vi "Prime BSI Set Get ROI.vi"(0 "Notifier In":refnum<notifier>, 5 "PVCam Actions":T3, 7 "Camera Ref":refnum<k24>, 11 "Error In":errorcluster, 13 "Image Ref":T1) -> (4 "Notifier Out":refnum<notifier>, 8 "PVCam Cluster":T2, 15 "Error Out":errorcluster)   [LabVIEW 2020]
uses:
  Prime BSI Type Defs/Prime BSI Actions.ctl
  C:/Users/Public/Documents/Photometrics/PMQI-LabViewSamples BETA/Examples/2020/Dependencies/PVCamNET.dll
  Public/Documents/Photometrics/PMQI-LabViewSamples BETA/Examples/2020/Dependencies/PVCamNET.dll
  Prime BSI Type Defs/Prime BSI Notifier Element.ctl
  Prime BSI Type Defs/Prime BSI Parameters.ctl
  Prime BSI Type Defs/Prime BSI Parameter List.ctl
  Prime BSI Type Defs/Prime BSI ROI.ctl
  <vilib>/vision/Image Controls.llb/IMAQ Image.ctl
  Camera Controls/Camera IMAQ Key Info.ctl
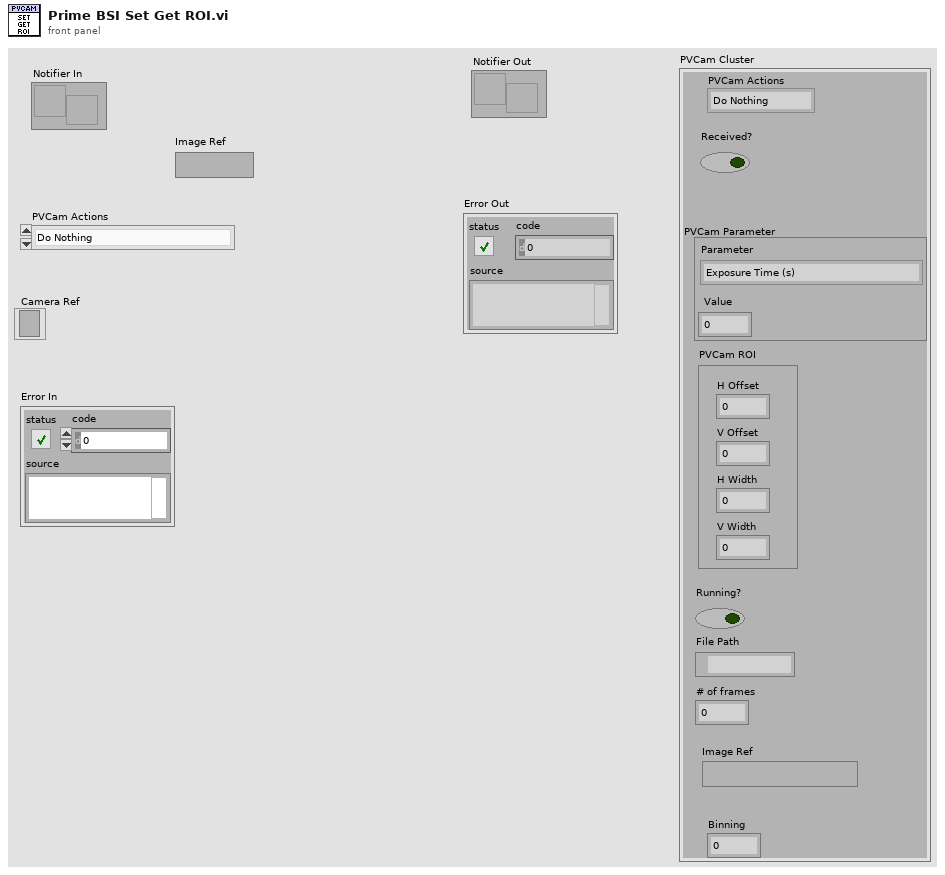
[diagram p1: front panel]
types:
  T1 = typedef "IMAQ Image.ctl" = refnum<image>
  T2 = typedef "Prime BSI Notifier Element.ctl" = cluster{"PVCam Actions":T3, "Received?":bool, "PVCam Parameter":T4, "PVCam ROI":T6, "Running?":bool, "File Path":path, "# of frames":u32, "Image Ref":T1, "Binning":i32}
  T3 = typedef "Prime BSI Actions.ctl" = enum16{"Do Nothing", "Preview", "Record", "Abort", "Record Settings", "Set Parameter", "Get Parameter", "Set ROI", "Get ROI", "Status", "Quit"}
  T4 = typedef "Prime BSI Parameters.ctl" = cluster{"Parameter":T5, "Value":dbl}
  T5 = typedef "Prime BSI Parameter List.ctl" = enum16{"Exposure Time (s)", "Binning"}
  T6 = typedef "Prime BSI ROI.ctl" = cluster{"H Offset":i32, "V Offset":i32, "H Width":i32, "V Width":i32}
  T7 = typedef "Camera IMAQ Key Info.ctl" = cluster{"Frame":u32, "Sensor Height":i32, "Sensor Width":i32, "ROI Height":i32, "ROI Width":i32, "ROI Enable?":bool, "Bit per Pixel":u8}
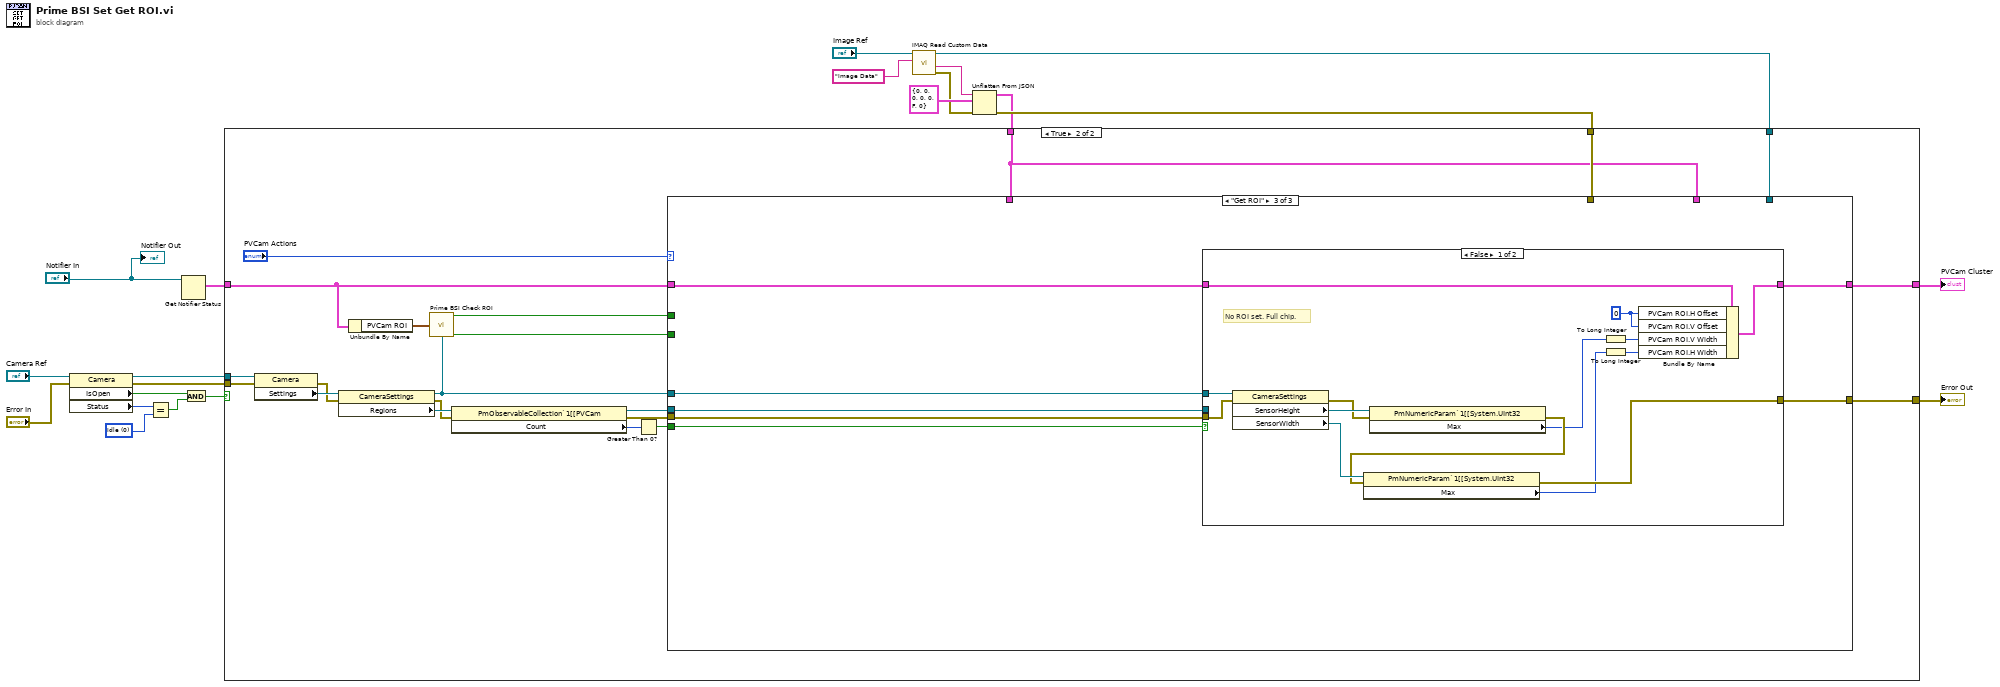
[diagram p0: block diagram]
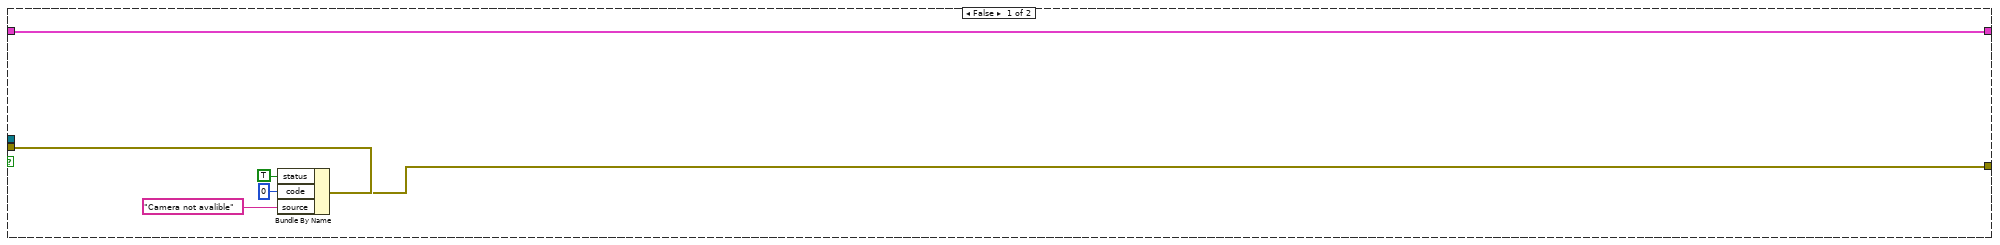
[diagram p2: hidden frame]
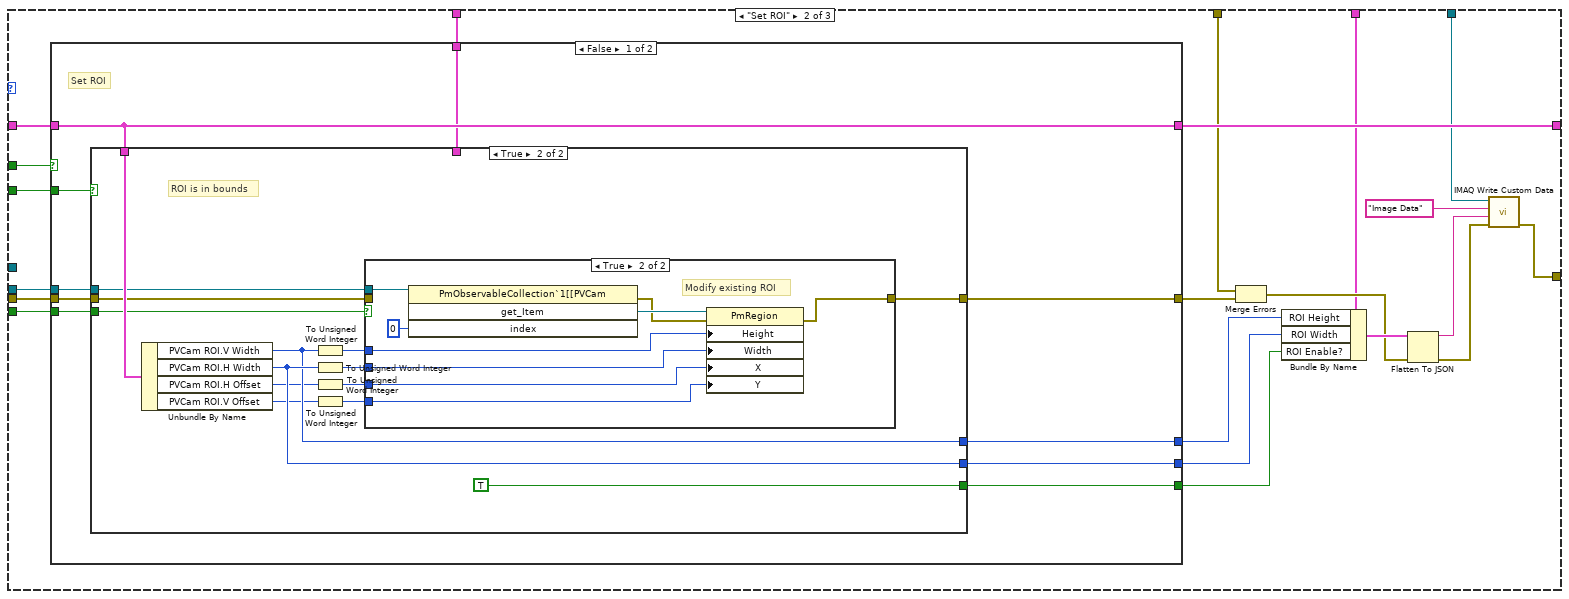
[diagram p4: hidden frame]
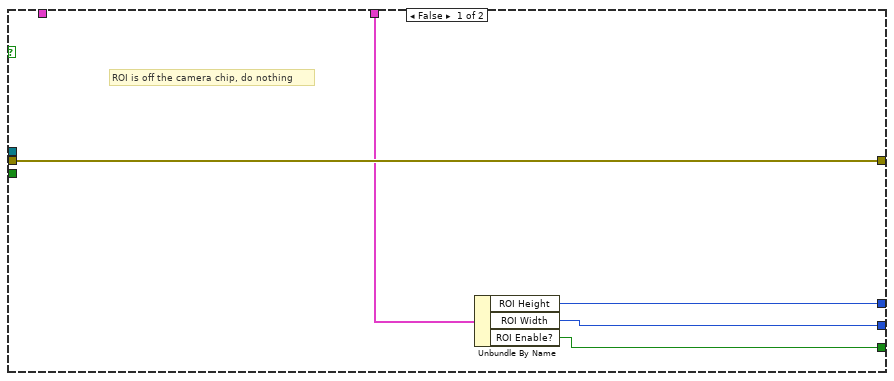
[diagram p5: hidden frame]
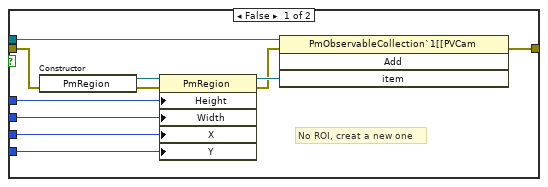
[diagram p6: hidden frame]
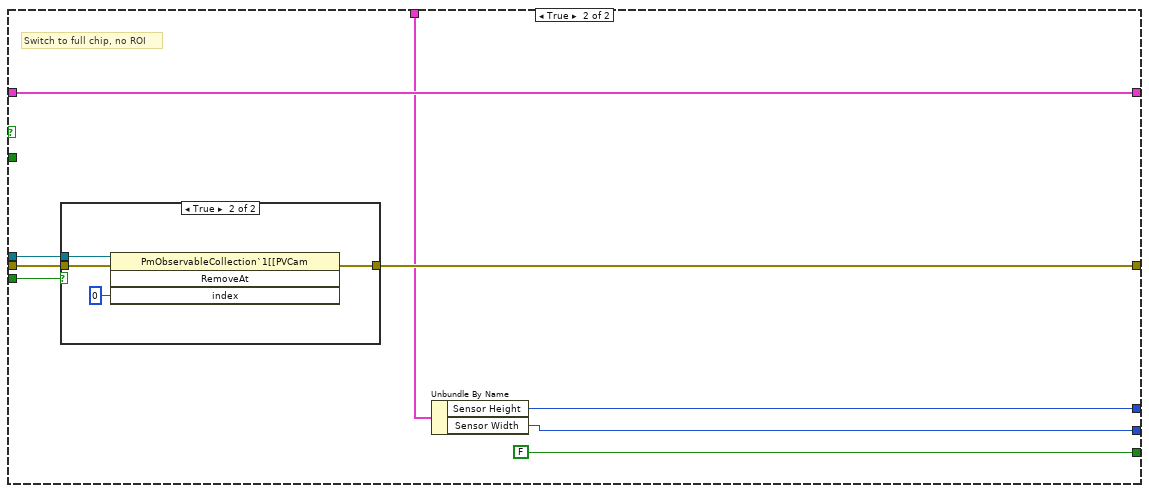
[diagram p7: hidden frame]
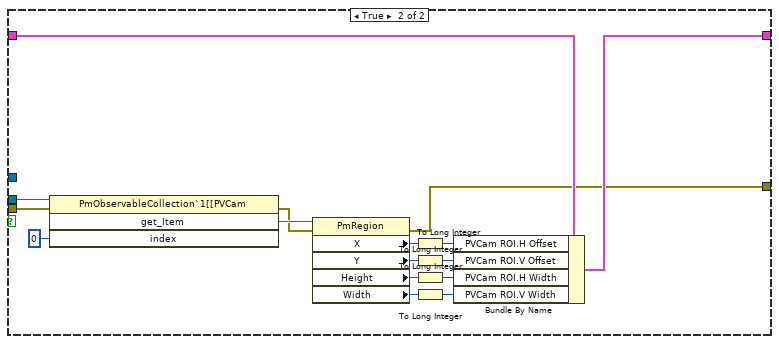
[diagram p9: hidden frame]
diagram:
  w20 = 0 items=["Idle", "Capturing"] ("Status")
  n1 = property class="Camera"(reference="Camera Ref", error in="Error In") -> (reference out=w14:refnum<k24>, error out=w13:errorcluster, "IsOpen"=w19:bool, "Status"=w21:i32)
  n2 = Equal?(x=w21, y=w20) -> (x = y?=w18:bool)
  n3 = Get Notifier Status(notifier="Notifier In") -> (current notification=w10:T2)  [unwired: 1 in, 4 out]
  n4 = And(x=w19, y=w18) -> (x .and. y?=w15:bool)
  n5 = call "IMAQ Read Custom Data"("Key"="Image Data", "Image"="Image Ref") -> ("error out"=w4:errorcluster, "Custom Data Out"=w6:string, "Image (duplicate)"=w3:T1)  [unwired: 7 in]
  n6 = Unflatten From JSON(JSON string=w6, type and defaults=T7 {"Frame"=0, "Sensor Height"=0, "Sensor Width"=0, "ROI Height"=0, "ROI Width"=0, "ROI Enable?"=FALSE, "Bit per Pixel"=0} ("Camera IMAQ Key Info"), error in (no error)=w4) -> (value=w1:T7, error out=w2:errorcluster)  [unwired: 4 in]
  n7 = case shown="True" w15 {
    tunnel: w14 -> [_ w48]
    tunnel: w13 -> [w27 w47]
    tunnel: [w23 w46] -> w12
    tunnel: [w22 w44] -> w11
    tunnel: w10 -> [w22 w41]
    tunnel: w3 -> [_ w40]
    tunnel: w2 -> [_ w39]
    tunnel: w1 -> [_ w37]
    frame False {
      n8 = Bundle By Name(cluster=w27, "status"=TRUE, "code"=0, "source"="Camera not avalible") -> (w23:errorcluster)
    }
    frame True {
      n9 = property class="Camera"(reference=w48, error in=w47) -> (error out=w42:errorcluster, "Settings"=w43:refnum<k24>)  [unwired: 1 out]
      n10 = property class="CameraSettings"(reference=w43, error in=w42) -> (reference out=w28:refnum<k24>, error out=w32:errorcluster, "Regions"=w33:refnum<k24>)
      n11 = Unbundle By Name(w41) -> ("PVCam ROI"=w38:T6)
      n12 = call "Prime BSI Check ROI.vi"("PVCam ROI"=w38, "Cam Settings Ref"=w28) -> ("Full Chip?"=w36:bool, "ROI In Bounds?"=w35:bool)  [unwired: 12 in]
      n13 = property class="PmObservableCollection`1[[PVCam"(reference=w33, error in=w32) -> (reference out=w29:refnum<k24>, error out=w30:errorcluster, "Count"=w34:i32)
      n14 = Greater Than 0?(x=w34) -> (x > 0?=w31:bool)
      n15 = case shown="\"Get ROI\"" "PVCam Actions" {
        tunnel: [w49 w66 w139] -> w46
        tunnel: w41 -> [w50 w70 w141]
        tunnel: [w50 w65 w140] -> w44
        tunnel: w36 -> [_ w71 _]
        tunnel: w40 -> [_ w61 _]
        tunnel: w39 -> [_ w58 _]
        tunnel: w37 -> [_ w56 _]
        tunnel: w37 -> [_ w55 _]
        tunnel: w35 -> [_ w54 _]
        tunnel: w31 -> [_ w51 w138]
        tunnel: w30 -> [w49 w53 w137]
        tunnel: w29 -> [_ w52 w136]
        tunnel: w28 -> [_ _ w135]
        frame Default {
        }
        frame "Set ROI" {
          n16 = case shown="False" w71 {
            tunnel: w51 -> [w73 w129]
            tunnel: w52 -> [w72 w128]
            tunnel: w53 -> [w74 w127]
            tunnel: [w81 w126] -> w59
            tunnel: w70 -> [w80 w124]
            tunnel: [w80 w124] -> w65
            tunnel: [w78 w122] -> w63
            tunnel: [w79 FALSE ("ROI Enable?")] -> w64
            tunnel: [w77 w121] -> w62
            tunnel: w56 -> [w75 w123]
            tunnel: w54 -> [w76 _]
            frame False {
              # "Set ROI"
              n17 = case shown="True" w76 {
                tunnel: w74 -> [w86 w88]
                tunnel: [w86 w87] -> w81
                tunnel: w80 -> [_ w100]
                tunnel: [w84 TRUE ("ROI Enable?")] -> w79
                tunnel: [w82 w98] -> w78
                tunnel: [w83 w97] -> w77
                tunnel: w75 -> [w85 _]
                tunnel: w73 -> [_ w90]
                tunnel: w72 -> [_ w89]
                frame False {
                  # "ROI is off the camera chip, do nothing"
                  n18 = Unbundle By Name(w85) -> ("ROI Height"=w83:i32, "ROI Width"=w82:i32, "ROI Enable?"=w84:bool)
                }
                frame True {
                  # "ROI is in bounds"
                  n19 = Unbundle By Name(w100) -> ("PVCam ROI.V Width"=w97:i32, "PVCam ROI.H Width"=w98:i32, "PVCam ROI.H Offset"=w96:i32, "PVCam ROI.V Offset"=w95:i32)
                  n20 = To Unsigned Word Integer(number=w97) -> (unsigned 16bit integer=w93:u16)
                  n21 = To Unsigned Word Integer(number=w98) -> (unsigned 16bit integer=w92:u16)
                  n22 = To Unsigned Word Integer(number=w96) -> (unsigned 16bit integer=w91:u16)
                  n23 = To Unsigned Word Integer(number=w95) -> (unsigned 16bit integer=w94:u16)
                  n24 = case shown="True" w90 {
                    tunnel: w94 -> [w110 w114]
                    tunnel: w93 -> [w109 w117]
                    tunnel: w92 -> [w108 w116]
                    tunnel: w91 -> [w107 w115]
                    tunnel: w89 -> [w106 w120]
                    tunnel: w88 -> [w104 _]
                    tunnel: [w101 w112] -> w87
                    frame False {
                      # "No ROI, creat a new one"
                      n25 = constructor class="PmRegion"(error in=w104) -> (reference out=w111:refnum<k24>, error out=w103:errorcluster)  [unwired: 2 in, 1 out]
                      n26 = property class="PmRegion"(reference=w111, error in=w103, "Height"=w109, "Width"=w108, "X"=w107, "Y"=w110) -> (reference out=w105:refnum<k24>, error out=w102:errorcluster)
                      n27 = invoke class="PmObservableCollection`1[[PVCam" method="Add"(reference=w106, error in=w102, "item"=w105) -> (error out=w101:errorcluster)  [unwired: 1 in, 3 out]
                    }
                    frame True {
                      # "Modify existing ROI"
                      n28 = invoke class="PmObservableCollection`1[[PVCam" method="get_Item"(reference=w120, "index"=0) -> (error out=w113:errorcluster, "get_Item"=w118:refnum<k24>)  [unwired: 2 in, 2 out]
                      n29 = property class="PmRegion"(reference=w118, error in=w113, "Height"=w117, "Width"=w116, "X"=w115, "Y"=w114) -> (error out=w112:errorcluster)  [unwired: 1 out]
                    }
                  }
                }
              }
            }
            frame True {
              # "Switch to full chip, no ROI"
              n30 = case shown="True" w129 {
                tunnel: w128 -> [_ w134]
                tunnel: w127 -> [w130 w133]
                tunnel: [w130 w131] -> w126
                frame False {
                }
                frame True {
                  n31 = invoke class="PmObservableCollection`1[[PVCam" method="RemoveAt"(reference=w134, error in=w133, "index"=0) -> (error out=w131:errorcluster)  [unwired: 1 in, 3 out]
                }
              }
              n32 = Unbundle By Name(w123) -> ("Sensor Height"=w121:i32, "Sensor Width"=w122:i32)
            }
          }
          n33 = Merge Errors(w58, w59) -> (w57:errorcluster)
          n34 = Bundle By Name(cluster=w55, "ROI Height"=w62, "ROI Width"=w63, "ROI Enable?"=w64) -> (w67:T7)
          n35 = Flatten To JSON(anything=w67, error in (no error)=w57) -> (JSON string=w68:string, 11:w69:errorcluster)  [unwired: 1 in]
          n36 = call "IMAQ Write Custom Data"("error in (no error)"=w69, "Custom Data In"=w68, "Key"="Image Data", "Image"=w61) -> ("error out"=w66:errorcluster)  [unwired: 6 in, 1 out]
        }
        frame "Get ROI" {
          n37 = case shown="False" w138 {
            tunnel: w136 -> [_ w171]
            tunnel: w137 -> [w152 w170]
            tunnel: w141 -> [w155 w166]
            tunnel: [w154 w157] -> w140
            tunnel: [w147 w156] -> w139
            tunnel: w135 -> [w153 _]
            frame False {
              w146 = 0 ("PVCam ROI.H Offset")
              # "No ROI set. Full chip."
              n38 = property class="CameraSettings"(reference=w153, error in=w152) -> (error out=w149:errorcluster, "SensorHeight"=w151:refnum<k24>, "SensorWidth"=w150:refnum<k24>)  [unwired: 1 out]
              n39 = property class="PmNumericParam`1[[System.UInt32"(reference=w151, error in=w149) -> (error out=w148:errorcluster, "Max"=w145:u32)  [unwired: 1 out]
              n40 = property class="PmNumericParam`1[[System.UInt32"(reference=w150, error in=w148) -> (error out=w147:errorcluster, "Max"=w144:u32)  [unwired: 1 out]
              n41 = To Long Integer(number=w145) -> (32bit integer=w143:i32)
              n42 = To Long Integer(number=w144) -> (32bit integer=w142:i32)
              n43 = Bundle By Name(cluster=w155, "PVCam ROI.H Offset"=w146, "PVCam ROI.V Offset"=w146, "PVCam ROI.V Width"=w143, "PVCam ROI.H Width"=w142) -> (w154:T2)
            }
            frame True {
              n44 = invoke class="PmObservableCollection`1[[PVCam" method="get_Item"(reference=w171, error in=w170, "index"=0) -> (error out=w167:errorcluster, "get_Item"=w168:refnum<k24>)  [unwired: 1 in, 2 out]
              n45 = property class="PmRegion"(reference=w168, error in=w167) -> (error out=w156:errorcluster, "X"=w165:u16, "Y"=w163:u16, "Height"=w162:u16, "Width"=w161:u16)  [unwired: 1 out]
              n46 = To Long Integer(number=w165) -> (32bit integer=w164:i32)
              n47 = To Long Integer(number=w163) -> (32bit integer=w160:i32)
              n48 = To Long Integer(number=w162) -> (32bit integer=w159:i32)
              n49 = To Long Integer(number=w161) -> (32bit integer=w158:i32)
              n50 = Bundle By Name(cluster=w166, "PVCam ROI.H Offset"=w164, "PVCam ROI.V Offset"=w160, "PVCam ROI.H Width"=w159, "PVCam ROI.V Width"=w158) -> (w157:T2)
            }
          }
        }
      }
    }
  }
  "Error Out" <- w12
  "PVCam Cluster" <- w11
  "Notifier Out" <- "Notifier In"
